vi "Register Event Handler.vi"(8 "error in (no error)":errorcluster {"code" format="%.0x"}, 9 "CallbackFunctionPointer":i64 format="%.0g", 10 "EventType (IviWarningEvent)":i32(ring) items=["IviWarningEvent", "ServiceRequestEvent"], 11 "instrument handle":refnum<k15>) -> (0 "error out":errorcluster {"code" format="%.0x"}, 3 "instrument handle out":refnum<k15>)   [LabVIEW 2020, in "Keysight DAQ970.lvlib"]
doc: "Registers a driver application event handler callback function to be called when the specified event type occurs."
uses:
  Keysight DAQ970.lvlib
  KtDAQ970.dll
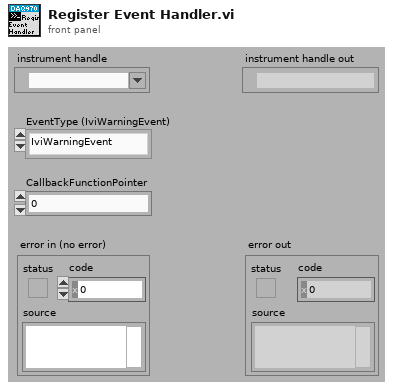
[diagram p1: front panel]
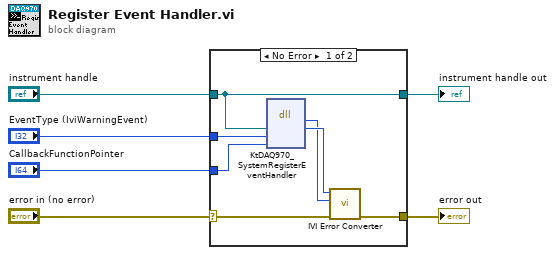
[diagram p0: block diagram]
diagram:
  n1 = case shown="No Error" "error in (no error)" {
    selector: "error in (no error)" -> [w11 w15]
    tunnel: [w10 w15] -> w6
    tunnel: "instrument handle" -> [w7 w14]
    tunnel: "EventType (IviWarningEvent)" -> [w9 _]
    tunnel: "CallbackFunctionPointer" -> [w8 _]
    tunnel: [w7 w14] -> w1
    frame No Error {
      n2 = dll-call lib="KtDAQ970**.dll" fn="KtDAQ970_SystemRegisterEventHandler"("Vi"=w7, "EventType"=w9, "CallbackFunctionPointer"=w8) -> ("return type"=w12:i32, "Vi"=w13:u32)  [unwired: 5 in, 2 out]
      n3 = call "IVI Error Converter.vi"("error in (no error)"=w11, "IVI error code (0)"=w12, "instrument handle"=w13) -> ("error out"=w10:errorcluster)  [unwired: 7 in, 1 out]
    }
    frame Error {
    }
  }
  "error out" <- w6
  "instrument handle out" <- w1
